vi "Call Counter.vi"(11 "Ref In":i32) -> (2 "Calls":i32, 3 "Ref Out":i32)   [LabVIEW 2013]
uses:
  Typedef/AI Table Node.ctl
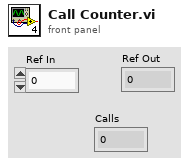
[diagram p1: front panel]
types:
  T1 = typedef "AI Table Node.ctl" = cluster{"Board State":i32, "Child Nodes":i32[], "X PCT":dbl, "O PCT":dbl, "Index":i32}
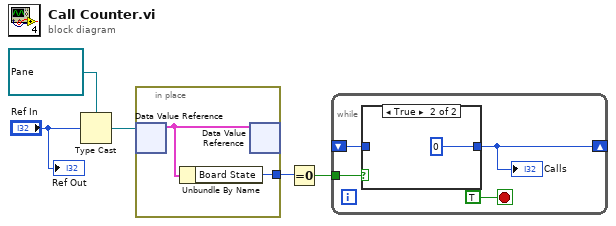
[diagram p0: block diagram]
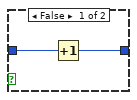
[diagram p2: hidden frame]
diagram:
  n1 = Type Cast(type=refnum<data-value> refnum ("data value reference"), x="Ref In") -> (*(type *) &x=w3:refnum<data-value>)
  n2 = in-place {
    in-place-border: [w6] -> w2
    n3 = in-place-dvr #1(w3) -> (w7:T1)  [unwired: 1 out]
    n4 = Unbundle By Name(w7) -> ("Board State"=w6:i32)
    n5 = in-place-dvr #1(w7) -> ()  [unwired: 2 out]
  }
  n6 = Equal To 0?(x=w2) -> (x = 0?=w1:bool)
  n7 = while {
    tunnel: w1 -> [w11]
    shift-right: [w9] -> _
    shift-left: _ -> [w8]
    stop <- TRUE stop-if-true
    n8 = case shown="True" w11 {
      tunnel: [w12 0] -> w9
      tunnel: w8 -> [w13 _]
      frame False {
        n9 = Increment(x=w13) -> (x+1=w12:i32)
      }
      frame True {
      }
    }
    "Calls" <- w9
  }
  "Ref Out" <- "Ref In"
